vi "Configure TS Panel.vi"(8 "error in":errorcluster, 11 "LNG Boiling Test Stand in":refnum<class "LNG Boiling Test Stand.lvclass">) -> (0 "error out":errorcluster, 3 "LNG Boiling Test Stand out":refnum<class "LNG Boiling Test Stand.lvclass">)   [LabVIEW 2019, in "Test Stands.lvlib" / "LNG Boiling Test Stand.lvclass"]
uses:
  LNG Boiling Test Stand.lvclass
  Generic Test Stand/Generic Test Stand.lvclass
  Results/LNG Boiling Results/LNG Boiling Results.lvclass
  C:/Users/krio/Documents/LV_Projects/test-stand/App/Generic Test Stand/Generic Test Stand.lvclass
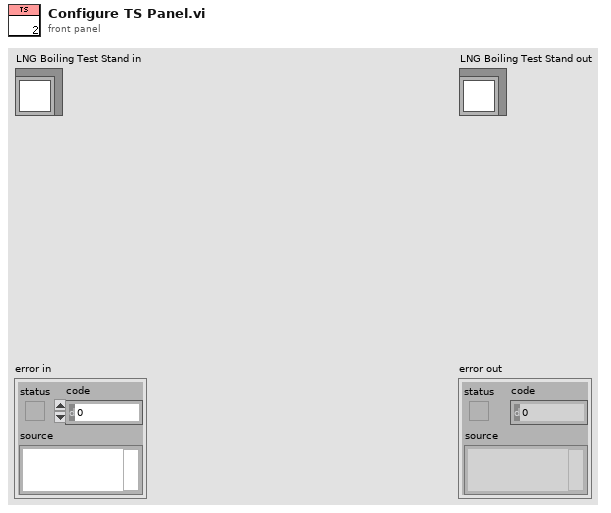
[diagram p1: front panel]
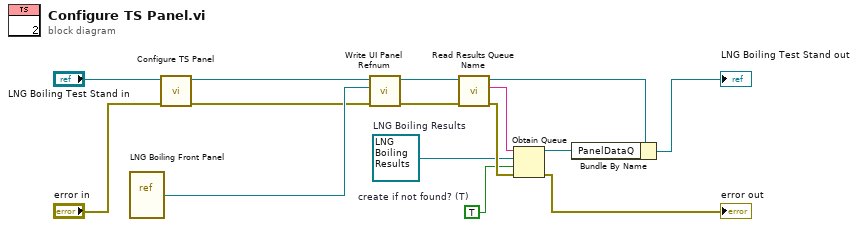
[diagram p0: block diagram]
diagram:
  w3 = TRUE  # create if not found? (T)
  w4 = refnum<class "LNG Boiling Results.lvclass"> refnum  # LNG Boiling Results
  n1 = vi-ref "LNG Boiling Front Panel.vi"() -> (w15:refnum<vi>)
  n2 = call-parent "Configure TS Panel.vi"("error in (no error)"="error in", "Generic Test Stand in"="LNG Boiling Test Stand in") -> ("error out"=w11:errorcluster, "Generic Test Stand out"=w13:refnum<class "LNG Boiling Test Stand.lvclass">)  [unwired: 8 in]
  n3 = call "Write UI Panel Refnum.vi"("error in (no error)"=w11, "UI Panel Refnum"=w15, "Generic Test Stand in"=w13) -> ("error out"=w7:errorcluster, "Generic Test Stand out"=w10:refnum<class "LNG Boiling Test Stand.lvclass">)  [unwired: 7 in]
  n4 = call "Read Results Queue Name.vi"("error in (no error)"=w7, "Generic Test Stand in"=w10) -> ("error out"=w5:errorcluster, "Results Queue Name"=w6:string, "Generic Test Stand out"=w9:refnum<class "LNG Boiling Test Stand.lvclass">)  [unwired: 7 in]
  n5 = Obtain Queue(name (unnamed)=w6, element data type=w4, create if not found? (T)=w3, error in (no error)=w5) -> (queue out=w2:refnum<queue>, error out=→"error out":errorcluster)  [unwired: 1 in, 1 out]
  n6 = Bundle By Name(cluster=w9, "PanelDataQ"=w2) -> (→"LNG Boiling Test Stand out":refnum<class "LNG Boiling Test Stand.lvclass">)
